vi "IMAQ_CoM_in_place_with_linefitting.vi"(4 "Destructive":bool, 6 "Inverted":bool, 7 "Optional Rectangle":i32[](array[numeric]), 8 "error in (no error)":errorcluster, 10 "background":u8, 11 "Image Src":T2) -> (0 "error out":errorcluster, 1 "Line Info":T1, 2 "Centroid":cluster{"X Centroid":sgl, "Y Centroid":sgl} {"Y Centroid" format="%.2f"; "X Centroid" format="%.2f"}, 3 "Image Src Dup":T2)   [LabVIEW 2010]
uses:
  <vilib>/vision/Image Controls.llb/IMAQ Image.ctl
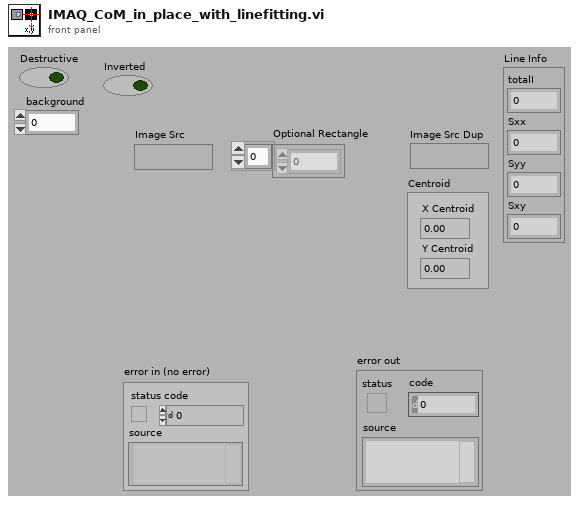
[diagram p1: front panel]
types:
  T1 = cluster{"totalI":sgl, "Sxx":sgl, "Syy":sgl, "Sxy":sgl}
  T2 = typedef "IMAQ Image.ctl" = refnum<image>
  T3 = enum32{"Map Pixel Pointer", "Unmap Pixel Pointer", "Get Pixels Infos"}
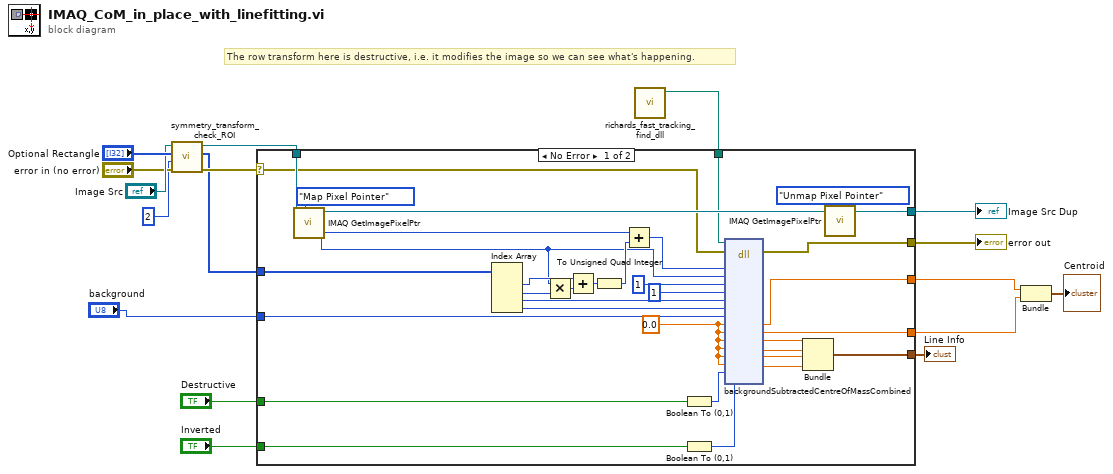
[diagram p0: block diagram]
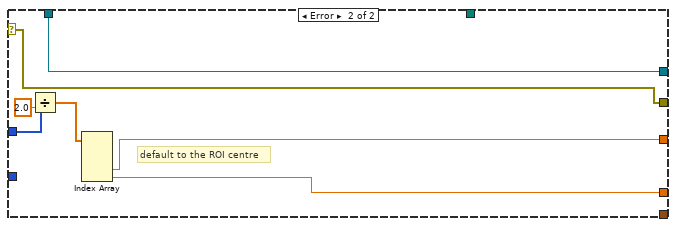
[diagram p2: hidden frame]
diagram:
  # "The row transform here is destructive, i.e. it modifies the image so we can see what's happening."
  n1 = call "symmetry_transform_check_ROI.vi"("error in (no error)"="error in (no error)", "minimum size"=2, "Optional Rectangle"="Optional Rectangle", "Image Src"="Image Src") -> ("error out"=w12:errorcluster, "ROI Out (x,y,w,h)"=w10:i32[], "Image Src Dup"=w13:T2)  [unwired: 1 in]
  n2 = call "richards_fast_tracking_find_dll.vi"() -> ("appended path"=w1:path)  [unwired: 11 in]
  n3 = case shown="No Error" w12 {
    selector: w12 -> [w32 w50]
    tunnel: [w29 w51] -> w9
    tunnel: [w28 w52] -> w8
    tunnel: w13 -> [w47 w56]
    tunnel: [w47 w56] -> w11
    tunnel: w10 -> [w34 w53]
    tunnel: "Destructive" -> [w21 _]
    tunnel: [w33 w50] -> w5
    tunnel: "background" -> [w31 _]
    tunnel: [w23 _] -> w3
    tunnel: "Inverted" -> [w20 _]
    tunnel: w1 -> [w18 _]
    frame No Error {
      w30 = sgl 0.0 ("CoMx")
      n4 = call "IMAQ GetImagePixelPtr"("Function"=T3."Map Pixel Pointer", "Image"=w47) -> ("LineWidth(Pixels)"=w36:i32, "Pixel Pointer out"=w35:u64)  [unwired: 4 in, 4 out]
      n5 = Index Array(array=w34) -> (element #1=w40:i32, element #2=w38:i32, element #3=w45:i32, element #4=w37:i32)  [unwired: 4 in]
      n6 = Multiply(x=w36, y=w38) -> (x*y=w39:i32)
      n7 = Add(x=w40, y=w39) -> (x+y=w41:i32)
      n8 = To Unsigned Quad Integer(1:w41) -> (0:w42:u64)
      n9 = Add(x=w35, y=w42) -> (x+y=w43:u64)
      n10 = Boolean To (0,1)(Boolean=w21) -> (0, 1=w22:i16)
      n11 = Boolean To (0,1)(Boolean=w20) -> (0, 1=w19:i16)
      n12 = dll-call lib="C:/Users/alinnenberger/Desktop/Cube/red_tweezers_1_4_rc0/RichardFastTracking/symmetrytransform32.dll" fn="backgroundSubtractedCentreOfMassCombined"(path in=w18, error in=w32, "pixelPointer"=w43, "skipx"=w36, "skipy"=1 ("LineWidth(Pixels)"), "pixelSizeInBytes"=1 ("LineWidth(Pixels)"), "width"=w45, "height"=w37, "background"=w31, "CoMx"=w30, "CoMy"=w30, "totalI"=w30, "Sxx"=w30, "Syy"=w30, "Sxy"=w30, "destructive"=w22, "inverted"=w19) -> (error out=w33:errorcluster, "CoMx"=w29:sgl, "CoMy"=w28:sgl, "totalI"=w24:sgl, "Sxx"=w25:sgl, "Syy"=w26:sgl, "Sxy"=w27:sgl)  [unwired: 11 in, 1 out]
      n13 = Bundle("totalI"=w24, "Sxx"=w25, "Syy"=w26, "Sxy"=w27) -> (w23:T1)  [unwired: 1 in]
      n14 = call "IMAQ GetImagePixelPtr"("Function"=T3."Unmap Pixel Pointer", "Image"=w47) -> ()  [unwired: 4 in, 6 out]
    }
    frame Error {
      # "default to the ROI centre"
      n15 = Divide(x=w53, y=2.0) -> (x/y=w55:dbl[])
      n16 = Index Array(array=w55) -> (element #3=w51:dbl, element #4=w52:dbl)  [unwired: 4 in, 2 out]
    }
  }
  "Image Src Dup" <- w11
  "error out" <- w5
  "Line Info" <- w3
  n17 = Bundle("CoMx"=w9, "CoMy"=w8) -> (→"Centroid":cluster{"CoMx":dbl, "CoMy":dbl})  [unwired: 1 out]
